vi "Peaprogramm.vi"() -> ()   [LabVIEW 2012]
panel:
  in  "Salvesta":bool
  in  "Graafik":bool
  in  "Kustuta":bool
  out "Vasak jalg 2":cluster{timestamp[], dbl[]}(graph)
  out "Parem jalg 2":cluster{timestamp[], dbl[]}(graph)
  in  "Filtreeri":bool
  out "Seade on leitud":bool=TRUE
  in  "Tühjenda nimekiri":bool
  in  "Vali kõik":bool
  out "Tehtud":bool
  in  "Valik":i32(listbox)
  in  "Alates (kellaaeg)":string="00:00"
  in  "Alates (kuupäev)":string="00.00.2010"
  in  "Kuni (kellaaeg)":string="22:22"
  in  "Kuni (kuupäev)":string="22.12.2013"
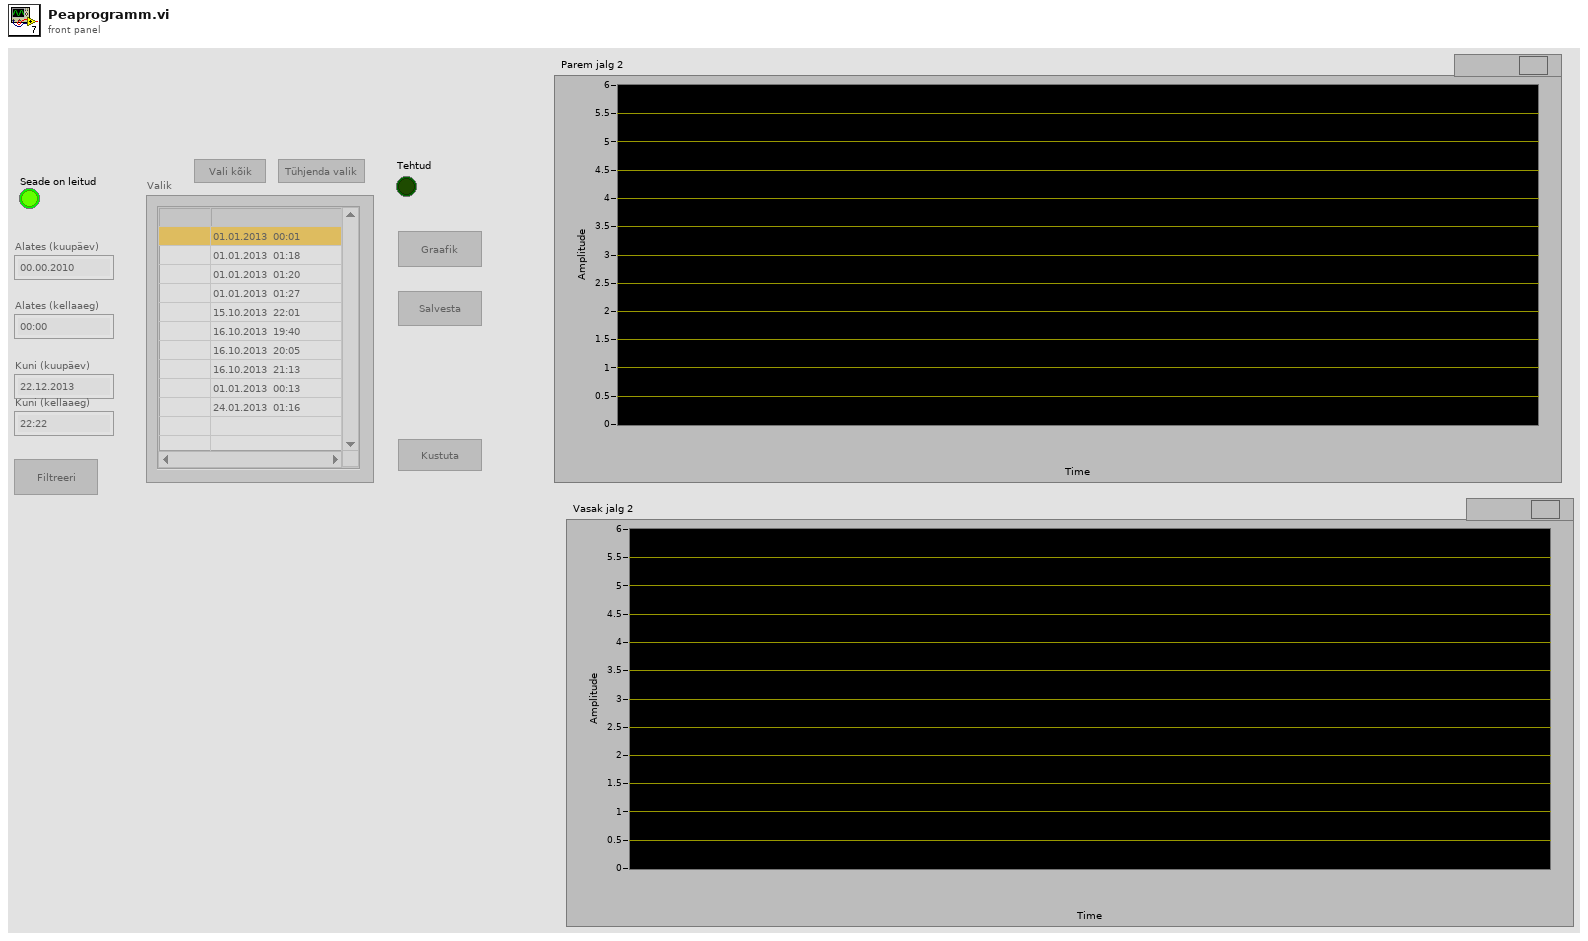
[diagram p1: front panel]
types:
  T1 = typedef "LVPoint32TypeDef.ctl" = cluster{"Horizontal":i32, "Vertical":i32}
  T2 = typedef "LVRowAndColumnTypeDef.ctl" = cluster{"Row":i32, "Column":i32}
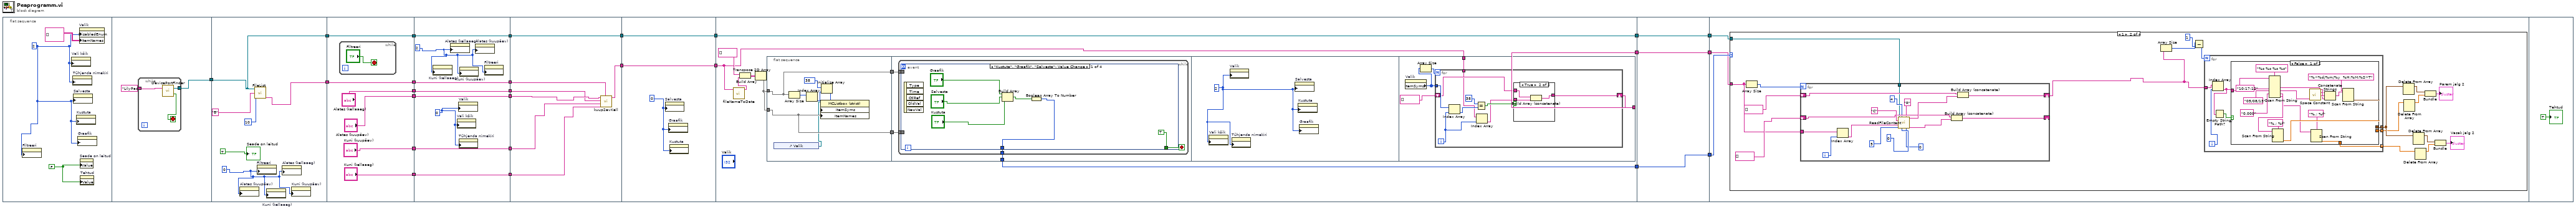
[diagram p0: block diagram]
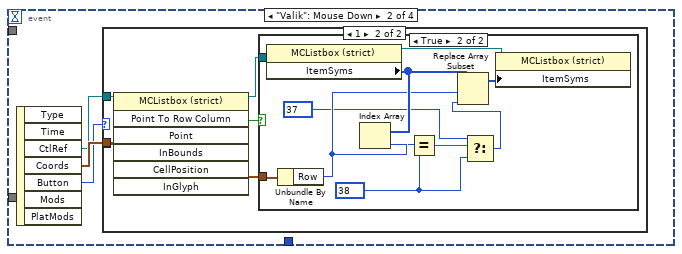
[diagram p2: hidden frame]
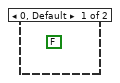
[diagram p3: hidden frame]
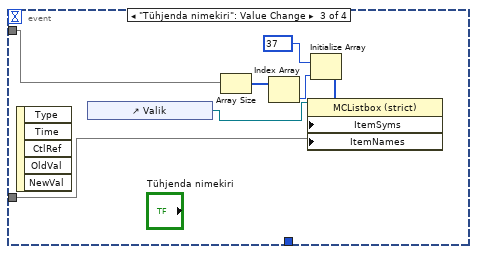
[diagram p5: hidden frame]
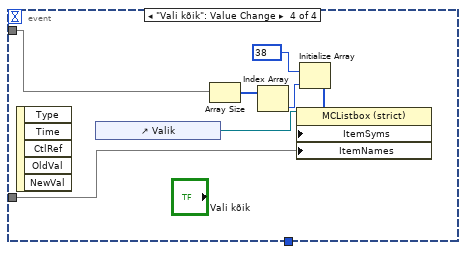
[diagram p6: hidden frame]
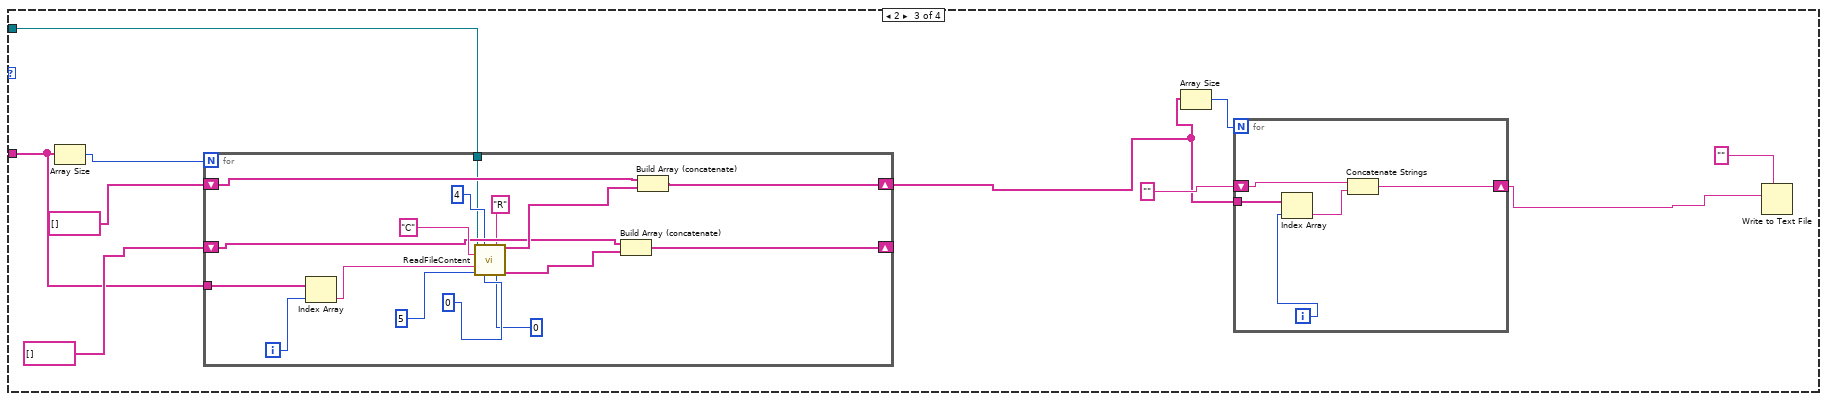
[diagram p10: hidden frame]
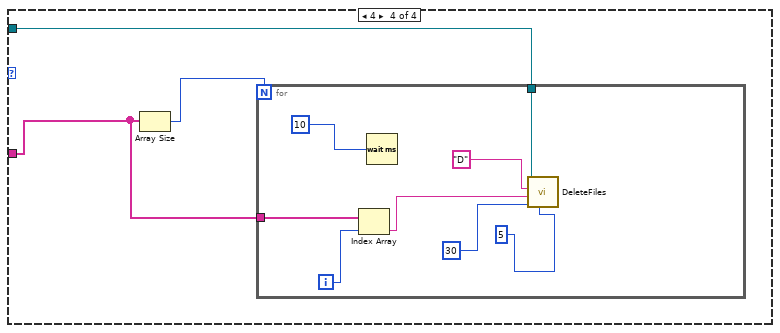
[diagram p11: hidden frame]
diagram:
  n1 = flat-sequence {
    tunnel: [w30] -> w25
    tunnel: [w36] -> w20
    tunnel: [w37] -> w19
    tunnel: w25 -> [w36]
    tunnel: w20 -> [w45]
    tunnel: [w45] -> w18
    tunnel: w19 -> [w44]
    tunnel: [w44] -> w16
    tunnel: ["Alates (kuupäev)"] -> w14
    tunnel: ["Alates (kellaaeg)"] -> w12
    tunnel: ["Kuni (kuupäev)"] -> w10
    tunnel: ["Kuni (kellaaeg)"] -> w8
    tunnel: w18 -> [w54]
    tunnel: [w54] -> w17
    tunnel: w16 -> [w53]
    tunnel: [w53] -> w15
    tunnel: w14 -> [w52]
    tunnel: [w52] -> w13
    tunnel: w12 -> [w51]
    tunnel: [w51] -> w11
    tunnel: w10 -> [w50]
    tunnel: [w50] -> w9
    tunnel: w8 -> [w49]
    tunnel: [w49] -> w7
    tunnel: w17 -> [w61]
    tunnel: [w61] -> w24
    tunnel: [w59] -> w22
    tunnel: w15 -> [w60]
    tunnel: w13 -> [w58]
    tunnel: w11 -> [w57]
    tunnel: w9 -> [w56]
    tunnel: w7 -> [w55]
    tunnel: w24 -> [w64]
    tunnel: [w64] -> w23
    tunnel: w22 -> [w63]
    tunnel: [w63] -> w21
    tunnel: w23 -> [w74]
    tunnel: [w74] -> w6
    tunnel: w21 -> [w68]
    tunnel: [w70] -> w5
    tunnel: [w65] -> w1
    tunnel: w6 -> [w149]
    tunnel: [w149] -> w4
    tunnel: w5 -> [w148]
    tunnel: [w148] -> w3
    tunnel: [w147] -> w2
    tunnel: w1 -> [w147]
    tunnel: w4 -> [w150]
    tunnel: w3 -> [w151]
    tunnel: w2 -> [w152]
    frame #0 {
      w26 = u8 2 ("Disabled")
      w28 = FALSE ("Valitud")
      n2 = property on="Filtreeri" class="Bool"("DisabledEnum"=w26) -> ()  [unwired: 2 in, 2 out]
      n3 = property on="Vali kõik" class="Bool"("DisabledEnum"=w26) -> ()  [unwired: 2 in, 2 out]
      n4 = property on="Tühjenda nimekiri" class="Bool"("DisabledEnum"=w26) -> ()  [unwired: 2 in, 2 out]
      n5 = property on="Salvesta" class="Bool"("DisabledEnum"=w26) -> ()  [unwired: 2 in, 2 out]
      n6 = property on="Kustuta" class="Bool"("DisabledEnum"=w26) -> ()  [unwired: 2 in, 2 out]
      n7 = property on="Graafik" class="Bool"("DisabledEnum"=w26) -> ()  [unwired: 2 in, 2 out]
      n8 = property on="Valik" class="MCListbox (strict)"("DisabledEnum"=w26, "ItemNames"=string[][] [] ("Item Names")) -> ()  [unwired: 2 in, 2 out]
      n9 = property on="Seade on leitud" class="Bool (strict)"("Value"=w28) -> ()  [unwired: 2 in, 2 out]
      n10 = property on="Tehtud" class="Bool (strict)"("Value"=w28) -> ()  [unwired: 2 in, 2 out]
    }
    frame #1 {
      n11 = while {
        tunnel: [w33] -> w30
        tunnel: "LilyPad" ("Substring") -> [w32]
        stop <- w31 stop-if-true
        n12 = call "DevicePortFinder.vi"("Substring"=w32) -> ("Port found"=w31:bool, "VISA resource name"=w33:refnum<visa-resource-name>)  [unwired: 1 in]
      }
    }
    frame #2 {
      w34 = u32 0 ("delay File List")
      n13 = property on="Alates (kuupäev)" class="Str"("DisabledEnum"=w34) -> ()  [unwired: 2 in, 2 out]
      n14 = call "FileList.vi"("VISA Refnum in"=w36, "delay File List"=u32 10, "string to write"="B") -> ("Array"=w37:string[])  [unwired: 12 in]
      n15 = property on="Filtreeri" class="Bool"("DisabledEnum"=w34) -> ()  [unwired: 2 in, 2 out]
      n16 = property on="Kuni (kellaaeg)" class="Str"("DisabledEnum"=w34) -> ()  [unwired: 2 in, 2 out]
      n17 = property on="Alates (kellaaeg)" class="Str"("DisabledEnum"=w34) -> ()  [unwired: 2 in, 2 out]
      n18 = property on="Kuni (kuupäev)" class="Str"("DisabledEnum"=w34) -> ()  [unwired: 2 in, 2 out]
      "Seade on leitud" <- TRUE ("Valitud")
    }
    frame #3 {
      n19 = while {
        stop <- "Filtreeri" stop-if-true
      }
    }
    frame #4 {
      w47 = u32 2 ("delay File List")
      w48 = u32 0 ("delay File List")
      n20 = property on="Kuni (kellaaeg)" class="Str"("DisabledEnum"=w47) -> ()  [unwired: 2 in, 2 out]
      n21 = property on="Alates (kellaaeg)" class="Str"("DisabledEnum"=w47) -> ()  [unwired: 2 in, 2 out]
      n22 = property on="Vali kõik" class="Bool"("DisabledEnum"=w48) -> ()  [unwired: 2 in, 2 out]
      n23 = property on="Valik" class="MCListbox (strict)"("DisabledEnum"=w48) -> ()  [unwired: 2 in, 2 out]
      n24 = property on="Tühjenda nimekiri" class="Bool"("DisabledEnum"=w48) -> ()  [unwired: 2 in, 2 out]
      n25 = property on="Kuni (kuupäev)" class="Str"("DisabledEnum"=w47) -> ()  [unwired: 2 in, 2 out]
      n26 = property on="Alates (kuupäev)" class="Str"("DisabledEnum"=w47) -> ()  [unwired: 2 in, 2 out]
      n27 = property on="Filtreeri" class="Bool"("DisabledEnum"=w47) -> ()  [unwired: 2 in, 2 out]
    }
    frame #5 {
      n28 = call "kuup2evKell.vi"("Sisend"=w60, "Kuni (kellaaeg)"=w55, "Kuni (kuupäev)"=w56, "Alates (kellaaeg)"=w57, "Alates (kuupäev)"=w58) -> ("V2ljund"=w59:string[])  [unwired: 5 in]
    }
    frame #6 {
      w62 = 0 ("x")
      n29 = property on="Salvesta" class="Bool"("DisabledEnum"=w62) -> ()  [unwired: 2 in, 2 out]
      n30 = property on="Graafik" class="Bool"("DisabledEnum"=w62) -> ()  [unwired: 2 in, 2 out]
      n31 = property on="Kustuta" class="Bool"("DisabledEnum"=w62) -> ()  [unwired: 2 in, 2 out]
    }
    frame #7 {
      n32 = call "fileNameToDate.vi"("Sisend"=w68) -> ("V2ljund"=w69:string[])  [unwired: 10 in]
      n33 = Build Array(string[] [] ("array"), w69) -> (w72:string[][])
      n34 = Transpose 2D Array(2D array=w72) -> (transposed array=w71:string[][])
      n35 = flat-sequence {
        tunnel: w71 -> [w77]
        tunnel: w71 -> [w76]
        tunnel: [w77] -> w67
        tunnel: [w76] -> w66
        tunnel: w67 -> [w84]
        tunnel: w66 -> [w83]
        tunnel: [w82] -> w65
        tunnel: [w131] -> w70
        tunnel: w68 -> [w129]
        frame #0 {
          n36 = control-ref of="Valik"() -> (w75:refnum<vi>)
          n37 = Array Size(array=w77) -> (size(s)=w81:i32[])
          n38 = Index Array(array=w81) -> (element=w79:i32)  [unwired: 1 in]
          n39 = Initialize Array(38, w79) -> (w80:i32[])
          n40 = property on="Property Node" class="MCListbox (strict)"(reference=w75, "ItemSyms"=w80, "ItemNames"=w76) -> ()  [unwired: 1 in, 2 out]
        }
        frame #1 {
          n41 = while {
            tunnel: w84 -> [w88]
            tunnel: w83 -> [w87]
            tunnel: [w86] -> w82
            stop <- w85 stop-if-true
            n42 = event shown="[0] \"Kustuta\", \"Graafik\", \"Salvesta\": Value Change" {
              selector: _ -> [_ _ _ _]
              dyn-events: _ -> [_ _ _ _]
              timeout: _ -> [_ _ _ _]
              tunnel: w88 -> [_ _ w116 w123]
              tunnel: w87 -> [_ _ w115 w122]
              tunnel: [w90 _ _ _] -> w86
              tunnel: [TRUE _ _ _] -> w85
              event "Kustuta", "Graafik", "Salvesta": Value Change {
                n43 = event-data() -> ()  [unwired: 1 in, 5 out]
                n44 = Build Array("Graafik", "Salvesta", "Kustuta") -> (w91:bool[])
                n45 = Boolean Array To Number(Boolean array=w91) -> (number=w90:u32)
              }
              event "Valik": Mouse Down {
                n46 = event-data() -> ("CtlRef"=w96:refnum<vi>, "Coords"=w97:T1, "Button"=w95:u16)  [unwired: 1 in, 4 out]
                n47 = case shown="1" w95 {
                  tunnel: [_ w100] -> _
                  tunnel: w97 -> [_ w100]
                  tunnel: w96 -> [_ w99]
                  frame 0, Default {
                    (unwired) FALSE
                  }
                  frame 1 {
                    n48 = invoke on="Invoke Node" class="MCListbox (strict)" method="Point To Row Column"(reference=w99, "Point"=w100) -> (reference out=w98:refnum<vi>, "CellPosition"=w102:T2, "InGlyph"=w101:bool)  [unwired: 5 in, 4 out]
                    n49 = case shown="True" w101 {
                      tunnel: w102 -> [_ w113]
                      tunnel: w98 -> [_ w111]
                      frame False {
                      }
                      frame True {
                        w105 = 38
                        n50 = property on="Property Node" class="MCListbox (strict)"(reference=w111) -> (reference out=w110:refnum<vi>, "ItemSyms"=w109:i32[])  [unwired: 1 in, 1 out]
                        n51 = Unbundle By Name(w113) -> ("Row"=w108:i32)
                        n52 = Index Array(array=w109, index=w108) -> (element=w107:i32)
                        n53 = Equal?(x=w107, y=w105) -> (x = y?=w106:bool)
                        n54 = Select(t=37, s=w106, f=w105) -> (s? t:f=w103:i32)
                        n55 = Replace Array Subset(array=w109, new element=w103, index=w108) -> (w112:i32[])
                        n56 = property on="Property Node" class="MCListbox (strict)"(reference=w110, "ItemSyms"=w112) -> ()  [unwired: 1 in, 2 out]
                      }
                    }
                  }
                }
              }
              event "Tühjenda nimekiri": Value Change {
                n57 = event-data() -> ()  [unwired: 1 in, 5 out]
                n58 = control-ref of="Valik"() -> (w114:refnum<vi>)
                n59 = Array Size(array=w116) -> (size(s)=w120:i32[])
                n60 = Index Array(array=w120) -> (element=w118:i32)  [unwired: 1 in]
                n61 = Initialize Array(37, w118) -> (w119:i32[])
                n62 = property on="Property Node" class="MCListbox (strict)"(reference=w114, "ItemSyms"=w119, "ItemNames"=w115) -> ()  [unwired: 1 in, 2 out]
              }
              event "Vali kõik": Value Change {
                n63 = event-data() -> ()  [unwired: 1 in, 5 out]
                n64 = control-ref of="Valik"() -> (w121:refnum<vi>)
                n65 = Array Size(array=w123) -> (size(s)=w127:i32[])
                n66 = Index Array(array=w127) -> (element=w125:i32)  [unwired: 1 in]
                n67 = Initialize Array(38, w125) -> (w126:i32[])
                n68 = property on="Property Node" class="MCListbox (strict)"(reference=w121, "ItemSyms"=w126, "ItemNames"=w122) -> ()  [unwired: 1 in, 2 out]
              }
            }
          }
        }
        frame #2 {
          w128 = 2 ("x")
          n69 = property on="Vali kõik" class="Bool"("DisabledEnum"=w128) -> ()  [unwired: 2 in, 2 out]
          n70 = property on="Valik" class="MCListbox (strict)"("DisabledEnum"=w128) -> ()  [unwired: 2 in, 2 out]
          n71 = property on="Tühjenda nimekiri" class="Bool"("DisabledEnum"=w128) -> ()  [unwired: 2 in, 2 out]
          n72 = property on="Salvesta" class="Bool"("DisabledEnum"=w128) -> ()  [unwired: 2 in, 2 out]
          n73 = property on="Kustuta" class="Bool"("DisabledEnum"=w128) -> ()  [unwired: 2 in, 2 out]
          n74 = property on="Graafik" class="Bool"("DisabledEnum"=w128) -> ()  [unwired: 2 in, 2 out]
        }
        frame #3 {
          n75 = property on="Valik" class="MCListbox (strict)"() -> ("ItemSyms"=w132:i32[])  [unwired: 2 in, 2 out]
          n76 = Array Size(array=w132) -> (size(s)=w133:i32)
          n77 = for {
            N: w133 -> [_]
            tunnel: w132 -> [w142]
            shift-right: [w137] -> w131
            shift-left: string[] [] -> [w138]
            tunnel: w129 -> [w136]
            i -> [w135]
            n78 = Index Array(array=w142, index=w135) -> (element=w141:i32)
            n79 = Equal?(x=38, y=w141) -> (x = y?=w139:bool)
            n80 = Index Array(array=w136, index=w135) -> (element=w134:string)
            n81 = case shown="True" w139 {
              tunnel: w138 -> [w143 w146]
              tunnel: [w143 w144] -> w137
              tunnel: w134 -> [_ w145]
              frame False {
              }
              frame True {
                n82 = Build Array (concatenate)(w146, w145) -> (w144:string[])
              }
            }
          }
        }
      }
    }
    frame #8 {
    }
    frame #9 {
      n83 = case shown="1" w152 {
        tunnel: w151 -> [_ w167 w217 w242]
        tunnel: w150 -> [_ w166 w216 w243]
        frame 0, Default {
        }
        frame 1 {
          n84 = Array Size(array=w167) -> (size(s)=w170:i32)
          n85 = for {
            N: w170 -> [_]
            shift-right: [w205] -> w154
            shift-left: string[] [] -> [w204]
            shift-right: [w202] -> _
            shift-left: string[] [] -> [w201]
            tunnel: w167 -> [w197]
            tunnel: w166 -> [w195]
            i -> [w210]
            n86 = Index Array(array=w197, index=w210) -> (element=w196:string)
            n87 = call "ReadFileContent.vi"("VISA Refnum in"=w195, "delay Data List"=u32 4, "File name string 2"="R", "Command String"="C", "File name string"=w196, "delay Input"=u32 5, "delay Command"=u32 0, "delay R"=u32 0) -> ("Array"=w206:string[], "Wrong"=w203:string[])  [unwired: 6 in]
            n88 = Build Array (concatenate)(w201, w203) -> (w202:string[])
            n89 = Build Array (concatenate)(w204, w206) -> (w205:string[])
          }
          n90 = Array Size(array=w154) -> (size(s)=w156:i32)
          n91 = Subtract(x=w156, y=1) -> (x-y=w155:i32)
          n92 = for {
            N: w155 -> [_]
            tunnel: w154 -> [w172]
            tunnel: [w176] -> w159 mode=indexing
            tunnel: [w175] -> w158 mode=indexing
            tunnel: [w174] -> w157 mode=indexing
            i -> [w171]
            n93 = Index Array(array=w172, index=w171) -> (element=w173:string)
            n94 = Empty String/Path?(string/path=w173) -> (empty?=w177:bool)
            n95 = case shown="False" w177 {
              tunnel: [w182 _] -> w175
              tunnel: [w181 _] -> w174
              tunnel: w173 -> [w183 _]
              tunnel: [w178 _] -> w176
              frame False {
                n96 = Scan From String(format string="%s %s %s %s", input string=w183, default 1="10:17:12", default 2="05/08/13", default 3="0.000") -> (output 1=w190:string, output 2=w189:string, output 3=w192:string, output 4=w179:string)  [unwired: 3 in, 3 out]
                n97 = Scan From String(format string="%.; %f", input string=w192) -> (output 1=w181:dbl)  [unwired: 3 in, 3 out]
                n98 = call <vilib>:"Space Constant.vi"() -> ("String"=w191:string)
                n99 = Scan From String(format string="%.; %f", input string=w179) -> (output 1=w178:dbl)  [unwired: 3 in, 3 out]
                n100 = Concatenate Strings(w189, w191, w190) -> (w187:string)
                n101 = Scan From String "Scan From String"(format string="%<%d/%m/%y  %H:%M:%S>T", input string=w187) -> (output 1=w182:timestamp)  [unwired: 3 in, 3 out]
              }
              frame True {
              }
            }
          }
          n102 = Delete From Array(array=w158) -> (array with subset deleted=w163:timestamp[])  [unwired: 2 in, 1 out]
          n103 = Delete From Array(array=w157) -> (array with subset deleted=w164:dbl[])  [unwired: 2 in, 1 out]
          n104 = Delete From Array(array=w158) -> (array with subset deleted=w160:timestamp[])  [unwired: 2 in, 1 out]
          n105 = Delete From Array(array=w159) -> (array with subset deleted=w161:dbl[])  [unwired: 2 in, 1 out]
          n106 = Bundle(w163, w164) -> (→"Parem jalg 2":cluster{timestamp[], dbl[]})  [unwired: 1 in]
          n107 = Bundle(w160, w161) -> (→"Vasak jalg 2":cluster{timestamp[], dbl[]})  [unwired: 1 in]
        }
        frame 2 {
          n108 = Array Size(array=w217) -> (size(s)=w220:i32)
          n109 = for {
            N: w220 -> [_]
            shift-right: [w236] -> w213
            shift-left: string[] [] -> [w235]
            shift-right: [w233] -> _
            shift-left: string[] [] -> [w232]
            tunnel: w217 -> [w228]
            tunnel: w216 -> [w226]
            i -> [w241]
            n110 = Index Array(array=w228, index=w241) -> (element=w227:string)
            n111 = call "ReadFileContent.vi"("VISA Refnum in"=w226, "delay Data List"=u32 4, "File name string 2"="R", "Command String"="C", "File name string"=w227, "delay Input"=u32 5, "delay Command"=u32 0, "delay R"=u32 0) -> ("Array"=w237:string[], "Wrong"=w234:string[])  [unwired: 6 in]
            n112 = Build Array (concatenate)(w232, w234) -> (w233:string[])
            n113 = Build Array (concatenate)(w235, w237) -> (w236:string[])
          }
          n114 = Array Size(array=w213) -> (size(s)=w215:i32)
          n115 = for {
            N: w215 -> [_]
            tunnel: w213 -> [w224]
            shift-right: [w222] -> w211
            shift-left: "" -> [w221]
            i -> [w225]
            n116 = Index Array(array=w224, index=w225) -> (element=w223:string)
            n117 = Concatenate Strings(w221, w223) -> (w222:string)
          }
          n118 = Write to Text File(prompt (Choose or enter file path)="", text=w211) -> ()  [unwired: 2 in, 3 out]
        }
        frame 4 {
          n119 = Array Size(array=w242) -> (size(s)=w244:i32)
          n120 = for {
            N: w244 -> [_]
            tunnel: w243 -> [w247]
            tunnel: w242 -> [w246]
            i -> [w252]
            n121 = Index Array(array=w246, index=w252) -> (element=w245:string)
            n122 = Wait (ms)(milliseconds to wait=u32 10 ("delay Per File Read")) -> ()  [unwired: 1 out]
            n123 = call "DeleteFiles.vi"("delay Command"=u32 5, "delay Input"=u32 30, "File name string"=w245, "Command String"="D", "VISA Refnum in"=w247) -> ()  [unwired: 7 in]
          }
        }
      }
    }
    frame #10 {
      "Tehtud" <- TRUE ("Kustutatud")
    }
  }
